vi "Send Configure Channel.vi"(7 "Message Priority (Normal)":T3=enum."Normal", 8 "error in (no error)":errorcluster, 10 "Settings":T1 {"Fall Time" format="%#_g s"; "Rise Time" format="%#_g s"; "Pulse Width" format="%#_g s"; "Symmetry" format="%#_g %"; "Phase" format="%#_g °"; "Offset" format="%#_g V"; "Amplitude" format="%#_g V"; "Frequency" format="%#_g Hz"}, 11 "Message Enqueuer":refnum<class "Message Enqueuer.lvclass">) -> (0 "error out":errorcluster, 3 "Message Enqueuer out":refnum<class "Message Enqueuer.lvclass">)   [LabVIEW 2019, in "FunctionGenerator.lvlib" / "Configure Channel Msg.lvclass"]
doc: "This VI sends the message to an actor."
uses:
  Configure Channel Msg.lvclass
  builds/Engine/Actor Framework.lvlibp/1abvi3w/vi.lib/ActorFramework/Message Enqueuer/Message Enqueuer.lvclass
  builds/Engine/Actor Framework.lvlibp/1abvi3w/vi.lib/ActorFramework/Message Enqueuer/Message Priority.ctl
  Custom Controls/WaveformSettings.ctl
  Custom Controls/WaveformMode.ctl
  Configure Channel Msg.lvclass/Configure Channel Msg.ctl
  C:/Users/Public/Documents/Development/builds/Engine/Actor Framework.lvlibp/1abvi3w/vi.lib/ActorFramework/Message/Message.lvclass
  Library/FunctionGenerator.lvclass
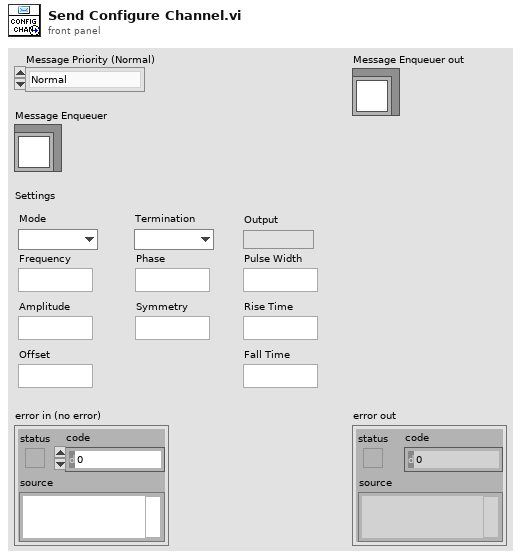
[diagram p1: front panel]
types:
  T1 = typedef "FunctionGenerator.lvlib/FunctionGenerator.lvclass/WaveformSettings.ctl" = cluster{"Frequency":dbl, "Amplitude":dbl, "Offset":dbl, "Phase":dbl, "Symmetry":dbl, "Pulse Width":dbl, "Rise Time":dbl, "Fall Time":dbl, "Mode":T2, "Termination":enum16{"50_Ohm", "High_Z"}, "Output":bool}
  T2 = typedef "FunctionGenerator.lvlib/FunctionGenerator.lvclass/WaveformMode.ctl" = enum16{"Sine", "Square", "Ramp", "Pulse", "Arbitrary", "Triangle", "Noise", "DC"}
  T3 = typedef "Actor Framework.lvlibp/Message Enqueuer.lvclass/Message Priority.ctl" = enum16{"Low", "Normal", "High"}
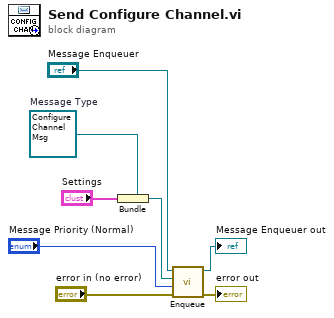
[diagram p0: block diagram]
diagram:
  w5 = refnum<class "Configure Channel Msg.lvclass"> refnum  # Message Type
  n1 = Bundle(cluster=w5, "Settings") -> (w4:refnum<class "Configure Channel Msg.lvclass">)
  n2 = call "Enqueue.vi"("error in (no error)"="error in (no error)", "Message Priority (Normal)"="Message Priority (Normal)", "Message"=w4, "Message Enqueuer in"="Message Enqueuer") -> ("error out"=→"error out":errorcluster, "Message Enqueuer out"=→"Message Enqueuer out":refnum<class "Message Enqueuer.lvclass">)  [unwired: 6 in]
